vi "AlliGator Decode PI Imaging Metadata Field.vi"(11 "Metadata Text Field":string) -> (1 "Metadata":string, 2 "Field":string)   [LabVIEW 2021, in "AlliGator Files.lvlib"]
doc: "Extract metadata from a Pi Imaging gate image field."
uses:
  AlliGator Files.lvlib
  <vilib>/Utility/error.llb/Error Cluster From Error Code.vi
  <vilib>/ErrorRing/Error Ring.xnode
panel:
  out "Error Out":errorcluster
  in  "Error In":errorcluster
  # "see the AlliGator License on the block diagram (Ctrl+E or Window:Show Block Diagram)"
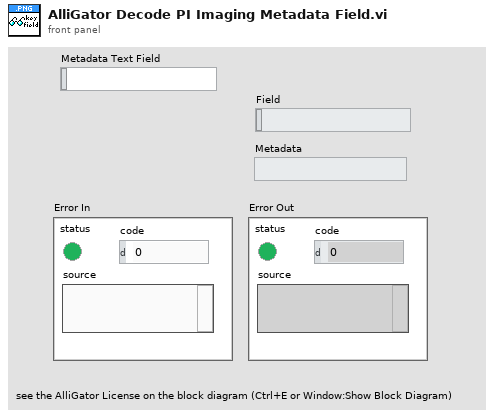
[diagram p1: front panel]
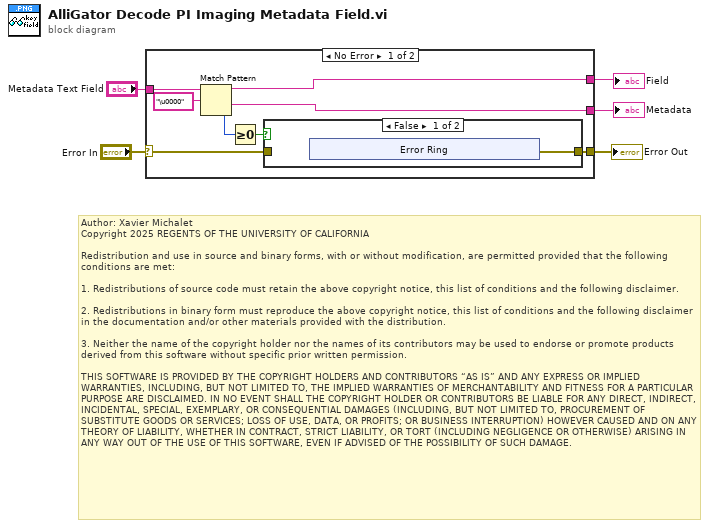
[diagram p0: block diagram]
diagram:
  # "Author: Xavier Michalet\nCopyright 2025 REGENTS OF THE UNIVERSITY OF CALIFORNIA\n\nRedistribution and use in source and binary forms, with or without modification, are permitted provided that the following conditions are met:\n\n1. Redistributions of source code must retain the above copyright notice, this list of conditions and the following disclaimer.\n\n2. Redistributions in binary form must reproduce the above copyright notice, this list of conditions and the following disclaimer in the documentation and/or other materials provided with the distribution.\n\n3. Neither the name of the copyright holder nor the names of its contributors may be used to endorse or promote products derived from this software without specific prior written permission.\n\nTHIS SOFTWARE IS PROVIDED BY THE COPYRIGHT HOLDERS AND CONTRIBUTORS “AS IS” AND ANY EXPRESS OR IMPLIED WARRANTIES, INCLUDING, BUT NOT LIMITED TO, THE IMPLIED WARRANTIES OF MERCHANTABILITY AND FITNESS FOR A PARTICULAR PURPOSE ARE DISCLAIMED. IN NO EVENT SHALL THE COPYRIGHT HOLDER OR CONTRIBUTORS BE LIABLE FOR ANY DIRECT, INDIRECT, INCIDENTAL, SPECIAL, EXEMPLARY, OR CONSEQUENTIAL DAMAGES (INCLUDING, BUT NOT LIMITED TO, PROCUREMENT OF SUBSTITUTE GOODS OR SERVICES; LOSS OF USE, DATA, OR PROFITS; OR BUSINESS INTERRUPTION) HOWEVER CAUSED AND ON ANY THEORY OF LIABILITY, WHETHER IN CONTRACT, STRICT LIABILITY, OR TORT (INCLUDING NEGLIGENCE OR OTHERWISE) ARISING IN ANY WAY OUT OF THE USE OF THIS SOFTWARE, EVEN IF ADVISED OF THE POSSIBILITY OF SUCH DAMAGE."
  n1 = case shown="No Error" "Error In" {
    selector: "Error In" -> [w7 w20]
    tunnel: [w13 _] -> w5
    tunnel: "Metadata Text Field" -> [w12 _]
    tunnel: [w9 _] -> w3
    tunnel: [w6 w20] -> w1
    frame No Error {
      n2 = Match Pattern(string=w12, regular expression="\u0000" ("String")) -> (before substring=w9:string, after substring=w13:string, offset past match=w10:i32)  [unwired: 1 in, 1 out]
      n3 = Greater Or Equal To 0?(x=w10) -> (x >= 0?=w8:bool)
      n4 = case shown="False" w8 {
        tunnel: w7 -> [_ w19]
        tunnel: [w14 w19] -> w6
        frame False {
          n5 = xnode "Error Ring"() -> ("error out"=w14:errorcluster)
        }
        frame True {
        }
      }
    }
    frame Error {
    }
  }
  "Metadata" <- w5
  "Field" <- w3
  "Error Out" <- w1
